vi "_Burn_EEPROM_vna_wmg.vi"(6 "Value":string, 8 "输出簇":T1={"seconds since 1Jan1904"=timestamp(3526253668.534785 s since 1904-01-01), "SNType"="LRyy(ddd)(X4)", "S/N:"="123", "SNNum"="4", "RS232 I2C VISA"="COM1", "Local Database"=FALSE, "命令类型选择"="LR Q to S 4X", "P/N:"="LM3QF001-SD-R"}) -> (0 "exist?":bool, 1 "字符串":string, 2 "cmd_input":string[][](array[string]), 3 "info_write":string[][](array[string]), 4 "legal":bool, 5 "readout":string[][](array[string]), 7 "type_array":string[](array[string]))   [LabVIEW 2011]
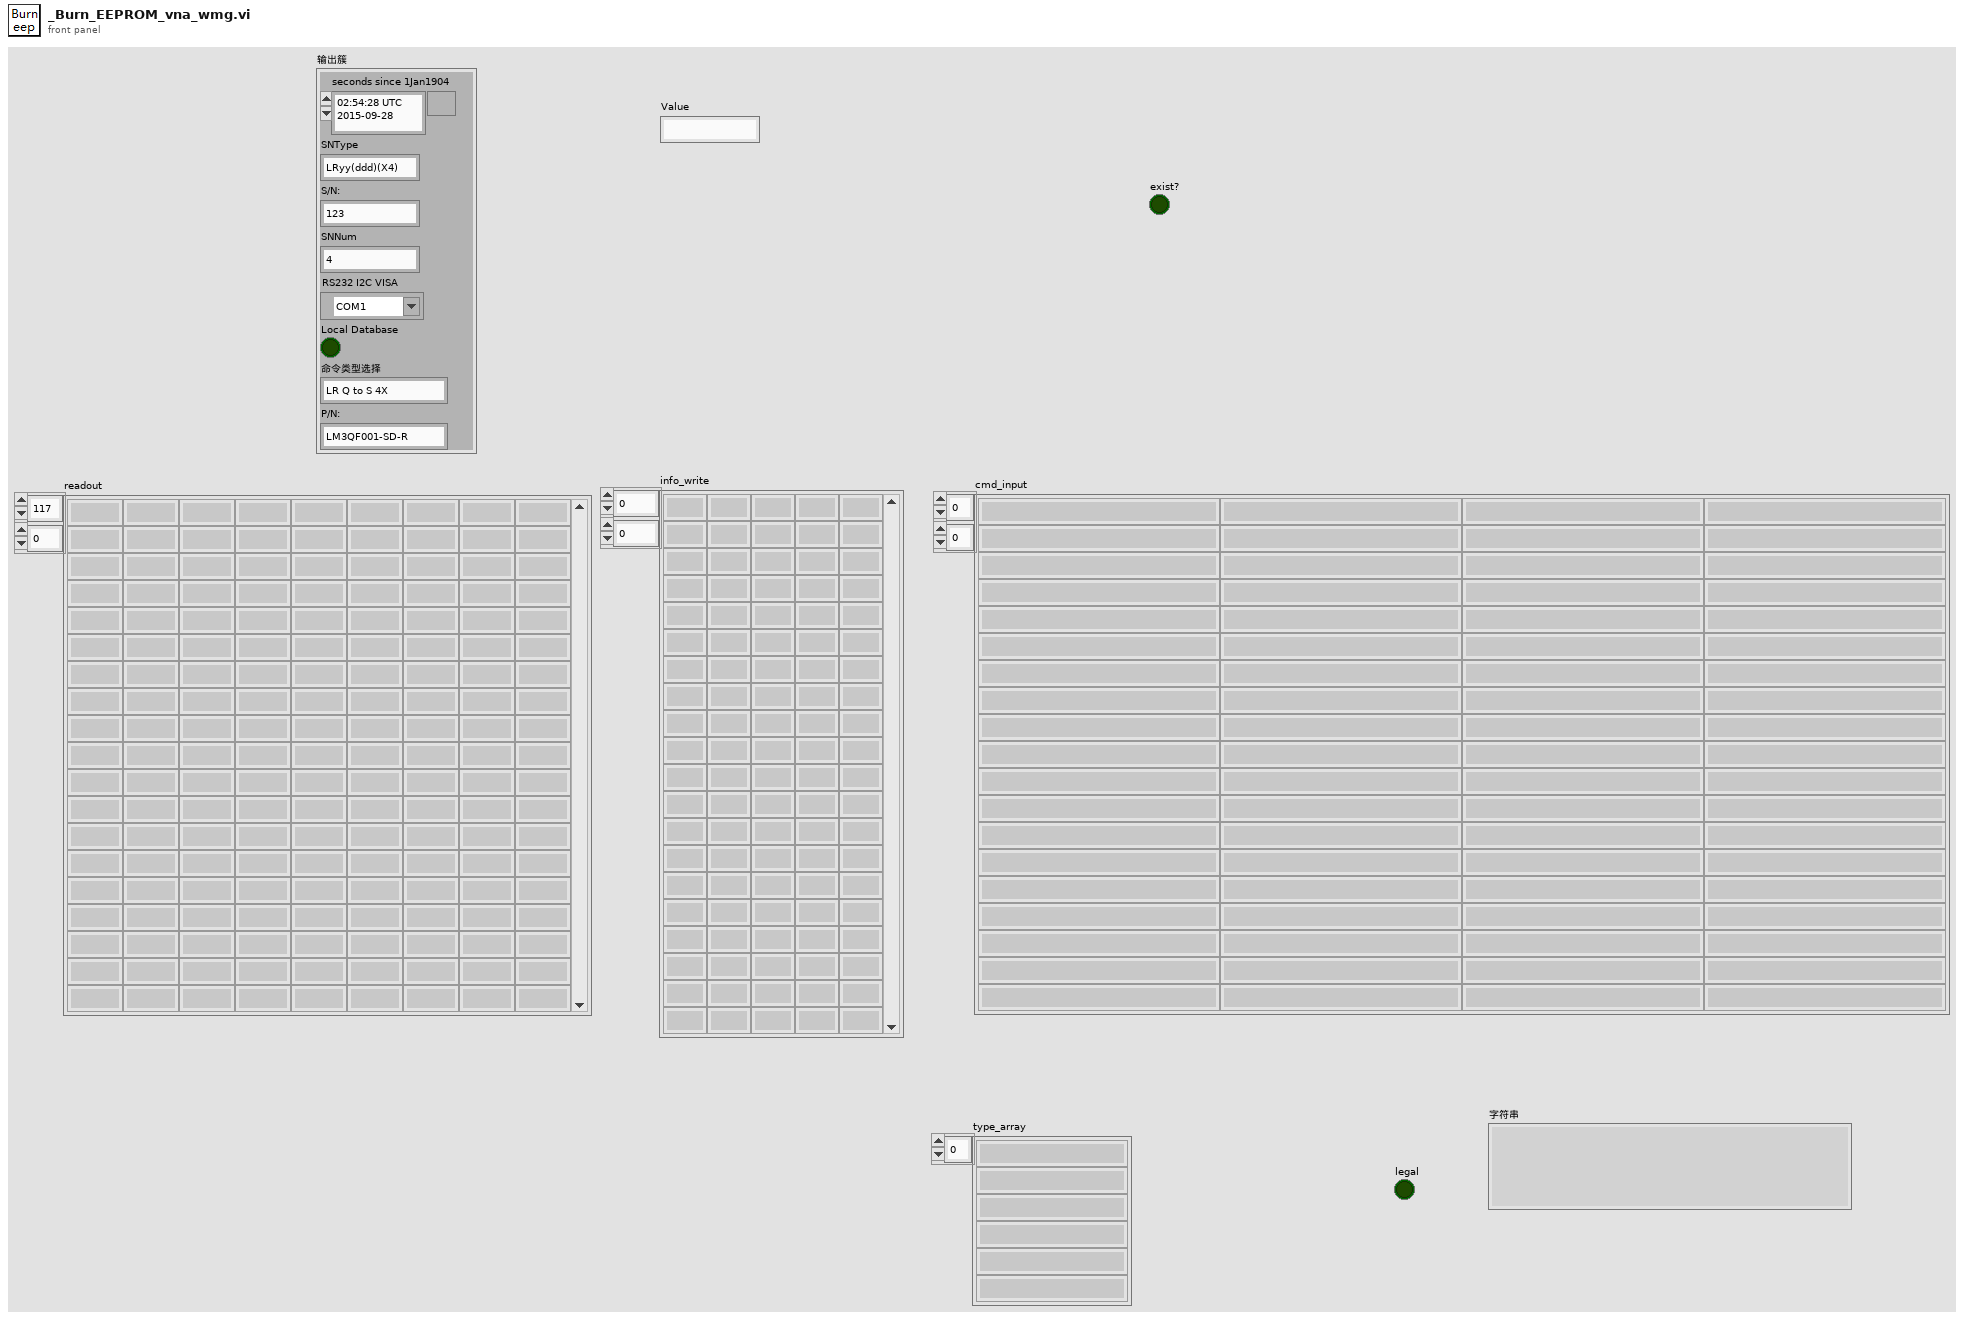
[diagram p1: front panel]
types:
  T1 = cluster{"seconds since 1Jan1904":timestamp, "SNType":string, "S/N:":string, "SNNum":string, "RS232 I2C VISA":refnum<visa-resource-name>, "Local Database":bool, "命令类型选择":string, "P/N:":string}
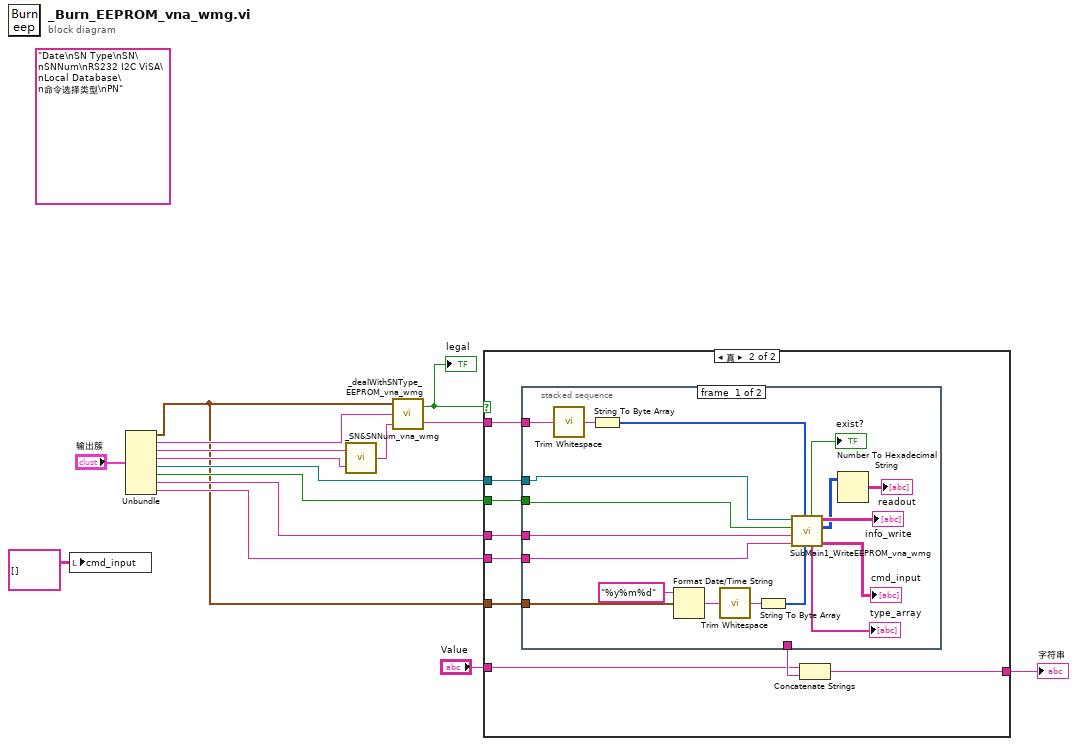
[diagram p0: block diagram]
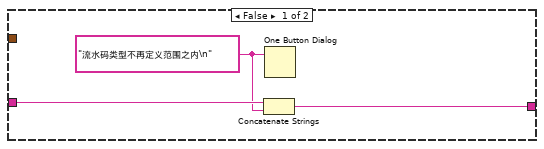
[diagram p2: hidden frame]
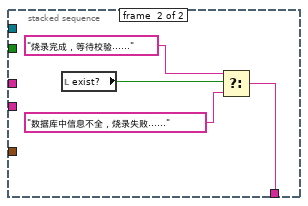
[diagram p3: hidden frame]
diagram:
  (unwired) "Date\nSN Type\nSN\nSNNum\nRS232 I2C ViSA\nLocal Database\n命令选择类型\nPN"
  n1 = local write "cmd_input"(string[][] [] ("cmd_input")) -> ()
  n2 = Unbundle("输出簇") -> ("seconds since 1Jan1904"=w4:timestamp, "SNType"=w11:string, "S/N:"=w10:string, "SNNum"=w9:string, "RS232 I2C VISA"=w8:refnum<visa-resource-name>, "Local Database"=w7:bool, "命令类型选择"=w6:string, "P/N:"=w5:string)
  n3 = call "_SN&SNNum_vna_wmg.vi"("SNNum"=w9, "SN"=w10) -> ("SN_out"=w13:string)
  n4 = call "_dealWithSNType_EEPROM_vna_wmg.vi"("SNXn"=w13, "SNType"=w11, "TimeInput"=w4) -> ("SNOutput"=w14:string, "legal"=w15:bool)
  "legal" <- w15
  n5 = case shown="真" w15 {
    tunnel: w14 -> [_ w27]
    tunnel: "Value" -> [w18 w24]
    tunnel: [w17 w26] -> w2
    tunnel: w8 -> [_ w23]
    tunnel: w7 -> [_ w22]
    tunnel: w6 -> [_ w21]
    tunnel: w5 -> [_ w20]
    tunnel: w4 -> [_ w19]
    frame False {
      w16 = "流水码类型不再定义范围之内\n" ("消息")
      n6 = Concatenate Strings(w18, w16) -> (w17:string)
      n7 = One Button Dialog(message=w16) -> ()  [unwired: 1 in, 1 out]
    }
    frame True {
      n8 = stacked-sequence {
        tunnel: w27 -> [w45 _]
        tunnel: [_ w46] -> w25
        tunnel: w23 -> [w33 _]
        tunnel: w22 -> [w32 _]
        tunnel: w21 -> [w31 _]
        tunnel: w20 -> [w30 _]
        tunnel: w19 -> [w29 _]
        frame #0 {
          n9 = call <vilib>:"Trim Whitespace.vi"("string"=w45) -> ("trimmed string"=w44:string)  [unwired: 1 in]
          n10 = String To Byte Array(string=w44) -> (unsigned byte array=w43:u8[])
          n11 = Format Date/Time String(time format string (%c)="%y%m%d" ("时间格式字符串(%c)"), seconds (now)=w29) -> (date/time string=w40:string)  [unwired: 1 in]
          n12 = call <vilib>:"Trim Whitespace.vi"("string"=w40) -> ("trimmed string"=w41:string)  [unwired: 1 in]
          n13 = String To Byte Array(string=w41) -> (unsigned byte array=w39:u8[])
          n14 = call "SubMain1_WriteEEPROM_vna_wmg.vi"("Date"=w39, "VendorSN"=w43, "PN"=w30, "命令类型选择"=w31, "local"=w32, "VISA resource name"=w33) -> ("cmd_input"=→"cmd_input":string[][], "readout"=w35:u8[][], "info_write"=→"info_write":string[][], "type_array"=→"type_array":string[], "exist?"=→"exist?":bool)  [unwired: 1 out]
          n15 = Number To Hexadecimal String(2:w35) -> (0:→"readout":string[][])  [unwired: 1 in]
        }
        frame #1 {
          n16 = local read "exist?"() -> (w49:bool)
          n17 = Select(t="烧录完成，等待校验......", s=w49, f="数据库中信息不全，烧录失败......") -> (s? t:f=w46:string)
        }
      }
      n18 = Concatenate Strings(w24, w25) -> (w26:string)
    }
  }
  "字符串" <- w2
